vi "GetType.vi"(8 "error in (no error)":errorcluster, 11 "Set Delay Msg":refnum<class "Set Delay Msg.lvclass">) -> (0 "error out":errorcluster, 2 "Data Sample":variant, 3 "Set Delay Msg":refnum<class "Set Delay Msg.lvclass">)   [LabVIEW 2021, in "BNT_ULx.lvlib" / "Set Delay Msg.lvclass"]
uses:
  Set Delay Msg.lvclass
  Set Delay Msg.lvclass/Set Delay Msg.ctl
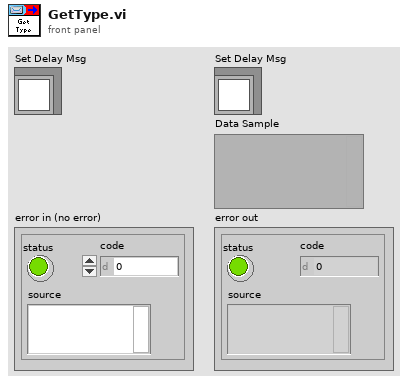
[diagram p1: front panel]
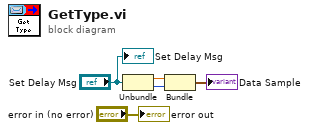
[diagram p0: block diagram]
diagram:
  n1 = Unbundle("Set Delay Msg") -> (w2:dbl, w1:i32)
  n2 = Bundle("PWM Delay"=w2, "Line"=w1) -> (→"Data Sample":cluster{"PWM Delay":dbl, "Line":i32})  [unwired: 1 in]
  "error out" <- "error in (no error)"
  "Set Delay Msg" <- "Set Delay Msg"
